vi "Setup Pulse Waveform.vi"(5 "Spacing":dbl=50.0, 7 "Delay":dbl=50.0, 8 "error in (no error)":errorcluster, 9 "Reset Pulse Conf":T1, 10 "Set Pulse Conf":T1, 11 "Actor_AFG in":refnum<class "Actor_AFG.lvclass">) -> (0 "error out":errorcluster, 3 "Actor_AFG out":refnum<class "Actor_AFG.lvclass">)   [LabVIEW 2020, in "Actor_AFG.lvlib" / "Actor_AFG.lvclass"]
uses:
  Actor_AFG.lvclass
  C:/Program Files/National Instruments/LabVIEW 2020/vi.lib/ActorFramework/Actor/Actor.lvclass
  AFG_Event.ctl
  Actor_AFG.lvclass/Actor_AFG.ctl
  <vilib>/ActorFramework/Actor/Actor.lvclass/Actor.ctl
  <instrlib>/Tektronix AFG 3000 Series/Tektronix AFG 3000 Series.lvlib
  <vilib>/ActorFramework/Actor/Actor.lvclass
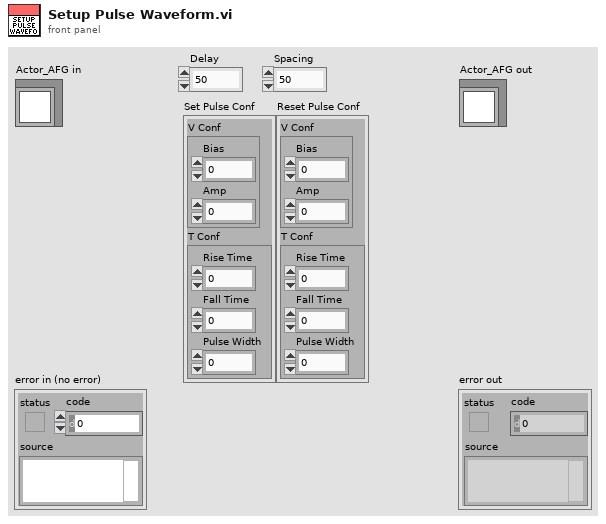
[diagram p1: front panel]
types:
  T1 = cluster{"V Conf":cluster{"Bias":dbl, "Amp":dbl}, "T Conf":cluster{"Rise Time":dbl, "Fall Time":dbl, "Pulse Width":dbl}}
  T2 = typedef "Actor_AFG.lvlib/Actor_AFG.lvclass/AFG_Event.ctl" = enum16{"General Event", "Inited", "Output", "Waveform Set", "Error"}
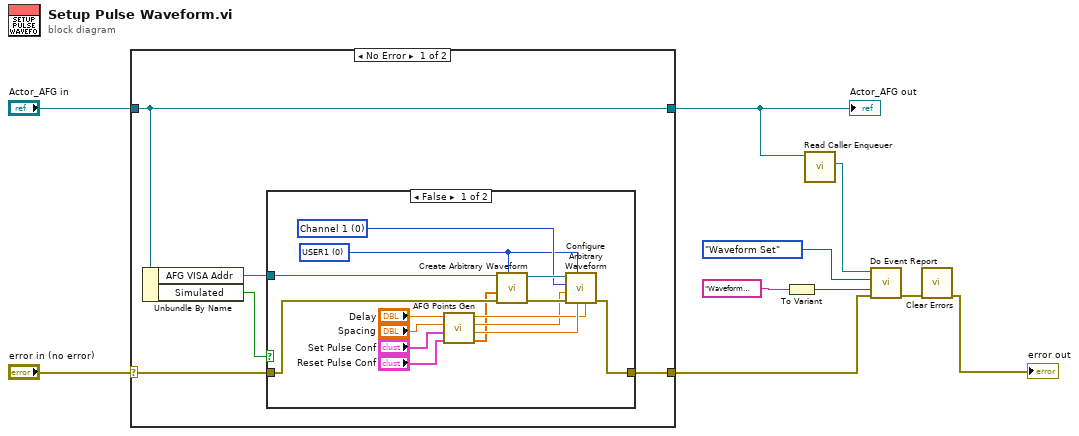
[diagram p0: block diagram]
diagram:
  n1 = case shown="No Error" "error in (no error)" {
    selector: "error in (no error)" -> [w15 w33]
    tunnel: [w11 w33] -> w4
    tunnel: [w12 w32] -> w8
    tunnel: "Actor_AFG in" -> [w12 w32]
    frame No Error {
      n2 = Unbundle By Name(w12) -> ("AFG VISA Addr"=w13:refnum<visa-resource-name>, "Simulated"=w14:bool)
      n3 = case shown="False" w14 {
        tunnel: w15 -> [w22 w31]
        tunnel: [w16 w31] -> w11
        tunnel: w13 -> [w26 _]
        frame False {
          w24 = u16 0 items=["Channel 1", "Channel 2"] ("Channel (0: Channel 1)")
          w23 = u16 0 items=["USER1", "USER2", "USER3", "USER4"] ("Arbitrary Waveform Name (0: USER1)")
          n4 = call "AFG Points Gen.vi"("Delay"="Delay", "Spacing"="Spacing", "Set Pulse Conf"="Set Pulse Conf", "Reset Pulse Conf"="Reset Pulse Conf") -> ("Frequency"=w19:dbl, "gain"=w18:dbl, "Offset"=w20:dbl, "Points Array"=w17:dbl[])  [unwired: 3 in]
          n5 = call <instrlib>:"Create Arbitrary Waveform.vi"("Arbitrary Waveform Name (0: USER1)"=w23, "error in (no error)"=w22, "Arbitrary Waveform Data"=w17, "VISA resource name"=w26) -> ("error out"=w21:errorcluster, "VISA resource name out"=w25:refnum<visa-resource-name>)  [unwired: 6 in]
          n6 = call <instrlib>:"Configure Arbitrary Waveform.vi"("Frequency (1000 Hz)"=w19, "DC Offset (0 V)"=w20, "Arbitrary Waveform Name (0: USER1)"=w23, "error in (no error)"=w21, "Gain (1 V)"=w18, "Channel (0: Channel 1)"=w24, "VISA resource name"=w25) -> ("error out"=w16:errorcluster)  [unwired: 3 in, 1 out]
        }
        frame True {
        }
      }
    }
    frame Error {
    }
  }
  "Actor_AFG out" <- w8
  n7 = To Variant(anything="Waveform Data Sent Successful") -> (Variant=w5:variant)
  n8 = call <vilib>:"Read Caller Enqueuer.vi"("Actor"=w8) -> ("Caller Enqueuer"=w1:refnum<class "Message Enqueuer.lvclass">)  [unwired: 10 in]
  n9 = call "Do Event Report.vi"("error in (no error)"=w4, "Event Data"=w5, "Report Events"=AFG_Event."Waveform Set", "Caller Enqueuer"=w1) -> ("error out"=w3:errorcluster)  [unwired: 6 in, 1 out]
  n10 = call <vilib>:"Clear Errors.vi"("error in (no error)"=w3) -> ("error out"=→"error out":errorcluster)  [unwired: 5 in, 1 out]
